vi "Emballage face avant pas de BDD.vi"() -> (0 "Annuler pb BDD":bool=TRUE, 1 "Qtté de la commande":string, 2 "DATA cmde":T1, 3 "N° cmde FAS":string)   [LabVIEW 2020]
panel:
  in  "Bouton Annuler":bool=TRUE
  # "Problème de connection\nà la base de données.\nLe programme va être arrêté."
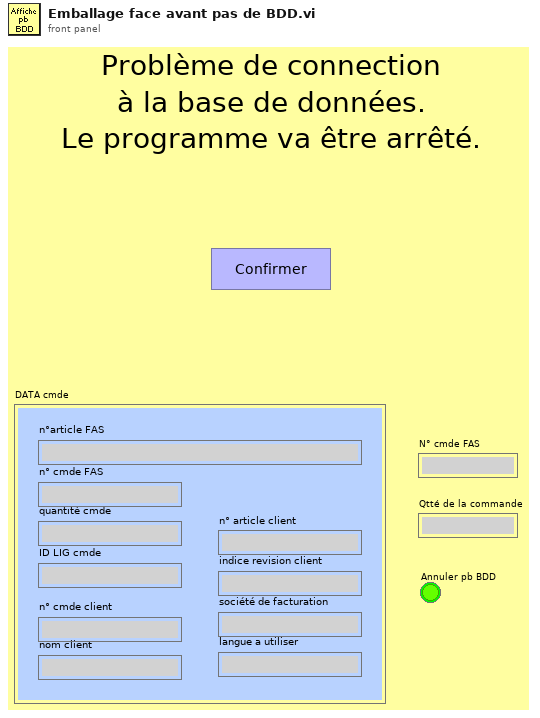
[diagram p1: front panel]
types:
  T1 = typedef "DATA commande.ctl" = cluster{"n°article FAS":string, "n° cmde FAS":string, "quantité cmde":string, "ID LIG cmde":string, "n° cmde client":string, "nom client":string, "n° article client":string, "indice revision client":string, "société de facturation":string, "langue a utiliser":string}
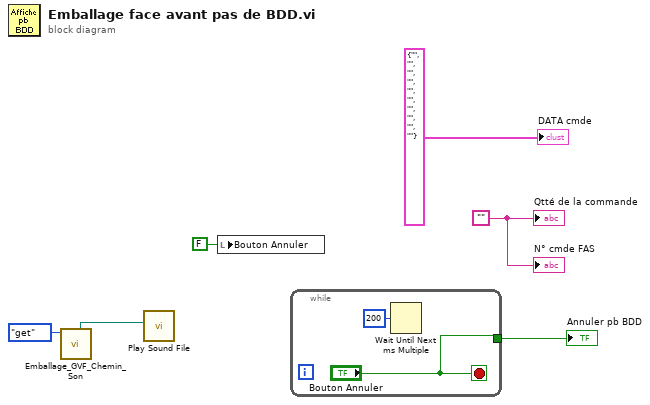
[diagram p0: block diagram]
diagram:
  w4 = ""
  n1 = call "Emballage_GVF_Chemin_Son.vi"("Énum"=enum16{"get", "set"}."get") -> ("Chemin Utopia - Erreur.WAV"=w2:path)  [unwired: 6 in, 4 out]
  n2 = call <vilib>:"Play Sound File.vi"("path"=w2) -> ()  [unwired: 9 in, 2 out]
  n3 = local write "Bouton Annuler"(FALSE) -> ()
  n4 = while {
    tunnel: ["Bouton Annuler"] -> w5
    stop <- "Bouton Annuler" stop-if-true
    n5 = Wait Until Next ms Multiple(millisecond multiple=200) -> ()  [unwired: 1 out]
  }
  "Annuler pb BDD" <- w5
  "Qtté de la commande" <- w4
  "N° cmde FAS" <- w4
  "DATA cmde" <- T1 {"n°article FAS"="", "n° cmde FAS"="", "quantité cmde"="", "ID LIG cmde"="", "n° cmde client"="", "nom client"="", "n° article client"="", "indice revision client"="", "société de facturation"="", "langue a utiliser"=""} ("DATA cmde")
